vi "State Queue PUSH multiple states no parameters.vi"(6 "Queue At Back? (T)":bool=TRUE, 7 "States to queue":string[](array[string]), 8 "error in (no error)":errorcluster, 11 "State que in":T1[](array[typedef])) -> (0 "error out":errorcluster, 3 "State que out":T1[](array[typedef]))   [LabVIEW 2013, in "State Machine Lib.lvlib"]
doc: "Pushes multiple states onto the stack, no parameters pushed here."
uses:
  State Machine Lib.lvlib
  STATE cluster.ctl
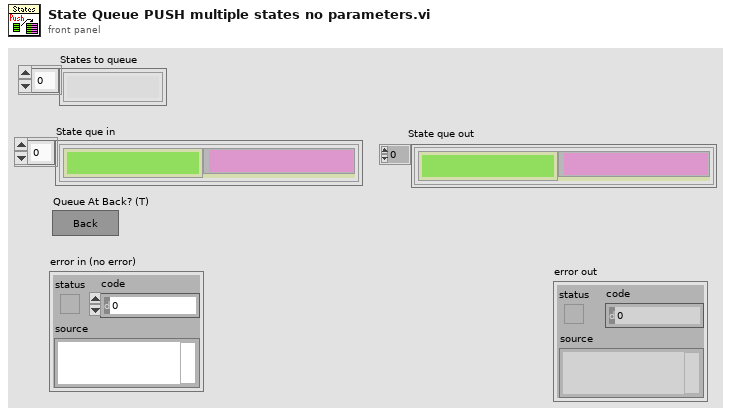
[diagram p1: front panel]
types:
  T1 = typedef "State Machine Lib.lvlib/STATE cluster.ctl" = cluster{"State":string, "Parameters":variant}
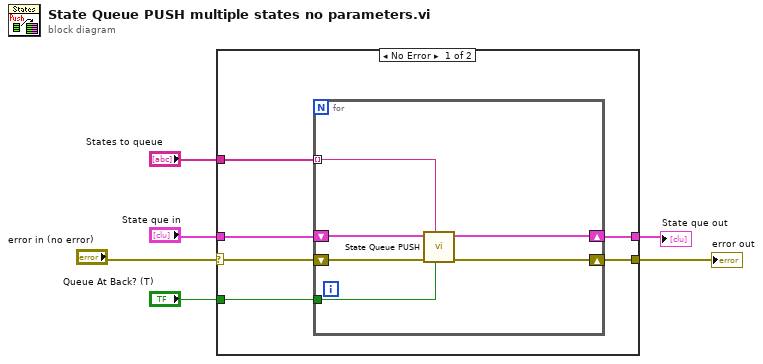
[diagram p0: block diagram]
diagram:
  n1 = case shown="No Error" "error in (no error)" {
    selector: "error in (no error)" -> [w11 w19]
    tunnel: [w11 w19] -> w6
    tunnel: "Queue At Back? (T)" -> [w10 _]
    tunnel: "States to queue" -> [w9 _]
    tunnel: [w8 w18] -> w2
    tunnel: "State que in" -> [w7 w18]
    frame No Error {
      n2 = for {
        shift-right: [w16] -> _
        shift-left: w11 -> [w17]
        tunnel: w10 -> [w15]
        shift-right: [w13] -> w8
        shift-left: w7 -> [w14]
        tunnel: w9 -> [w12] mode=indexing
        n3 = call "State Queue PUSH.vi"("Queue At Back? (T)"=w15, "State case"=w12, "error in (no error)"=w17, "State que in"=w14) -> ("error out"=w16:errorcluster, "State que out"=w13:T1[])  [unwired: 1 in, 5 out]
      }
    }
    frame Error {
    }
  }
  "State que out" <- w2
  "error out" <- w6
